vi "File.Filter SubDirs by DateName Range.vi"(10 "From_To":string[](array[string]), 11 "RootDir":path) -> (3 "SubDirs":path[](array[path]))   [LabVIEW 2019]
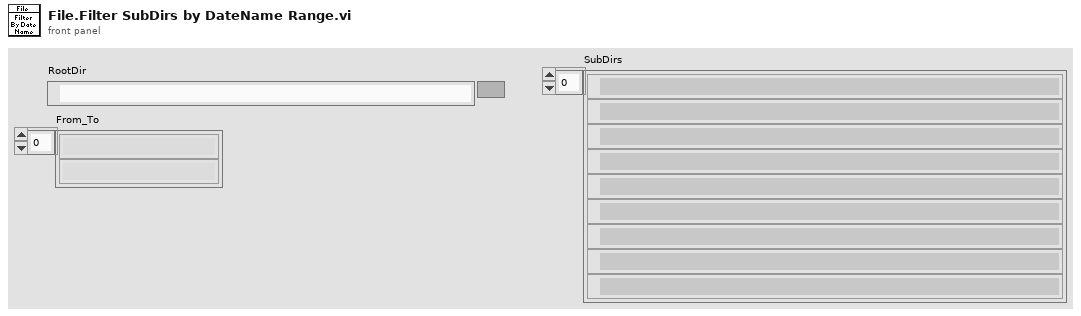
[diagram p1: front panel]
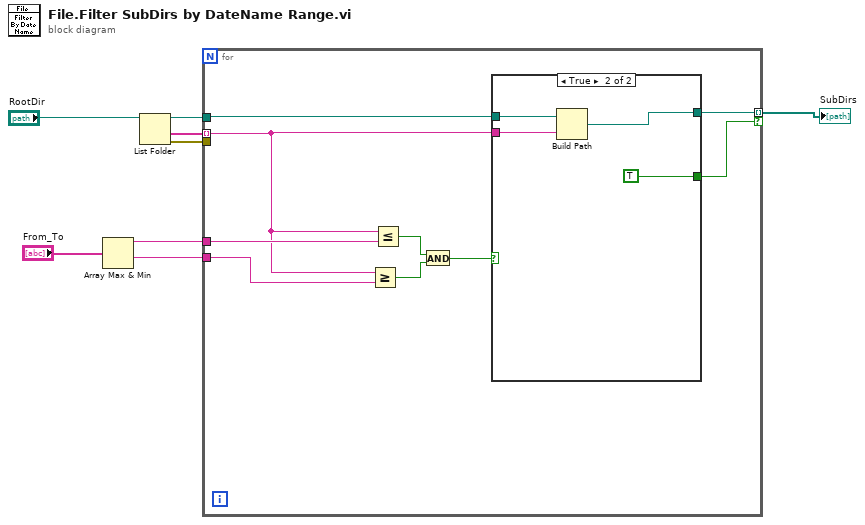
[diagram p0: block diagram]
diagram:
  n1 = Array Max & Min(array="From_To") -> (max value=w4:string, min value=w3:string)  [unwired: 2 out]
  n2 = List Folder(path="RootDir") -> (path out=w7:path, folder names=w6:string[], error out=w1:errorcluster)  [unwired: 3 in, 1 out]
  n3 = for {
    tunnel: w7 -> [w13]
    tunnel: w6 -> [w12] mode=indexing
    tunnel: w4 -> [w16]
    tunnel: w3 -> [w17]
    tunnel: [w10] -> w2 mode=indexing if=w9
    tunnel: w1 -> [_]
    n4 = Greater Or Equal?(x=w12, y=w17) -> (x >= y?=w14:bool)
    n5 = Less Or Equal?(x=w12, y=w16) -> (x <= y?=w15:bool)
    n6 = And(x=w15, y=w14) -> (x .and. y?=w11:bool)
    n7 = case shown="True" w11 {
      tunnel: w13 -> [_ w21]
      tunnel: w12 -> [_ w20]
      tunnel: [_ w19] -> w10
      tunnel: [_ TRUE] -> w9
      frame False {
      }
      frame True {
        n8 = Build Path(base path=w21, name or relative path=w20) -> (appended path=w19:path)
      }
    }
  }
  "SubDirs" <- w2
